vi "ros1.vi"() -> ()   [LabVIEW 2015]
uses:
  <vilib>/Tufts CEEO ROS for LabVIEW Software/ROS/Code/Console/Servers/ServerSubs/TopicDef.ctl
  <vilib>/Tufts CEEO ROS for LabVIEW Software/ROS/Code/SubVIs/_ROSDirection.ctl
  <vilib>/Tufts CEEO ROS for LabVIEW Software/ROS/MessageParsing/std_msgs/subs/parse_bool_scalar.vi
panel:
  out "bool":bool
  in  "Definitions":T1={"Topic"="/robot/head/command_head_nod", "Type"="std_msgs/Bool", "Action"=enum."Publisher", "Update (ms)"=1, "queue size"=1}
  in  "node":string
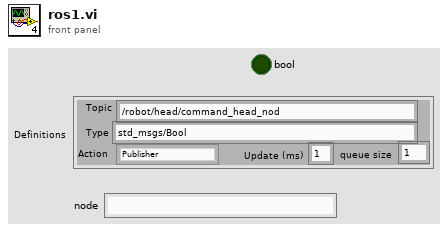
[diagram p1: front panel]
types:
  T1 = typedef "TopicDef.ctl" = cluster{"Topic":string, "Type":string, "Action":T2, "Update (ms)":u16, "queue size":u16}
  T2 = typedef "_ROSDirection.ctl" = enum16{"Node", "Publisher", "Subscriber", "ServiceClient", "ServiceProvider"}
  T3 = typedef "_ROSControl.ctl" = cluster{"topic port":u16, "Node":string, "topic":string, "type":string, "node port":u16, "error ":errorcluster, "Direction":T2, "Update (ms)":u16, "FIFO size":u16}
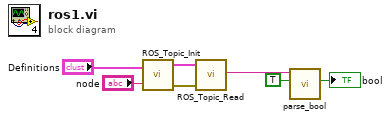
[diagram p0: block diagram]
diagram:
  n1 = call <vilib>:"ROS_Topic_Init.vi"("Definitions"="Definitions", "node"="node") -> ("ROS out"=w4:T3, "error out"=w5:errorcluster)  [unwired: 1 in]
  n2 = call <vilib>:"ROS_Topic_Read.vi"("error in (no error)"=w5, "ROS in"=w4) -> ("Reply"=w3:string)  [unwired: 1 in, 2 out]
  n3 = call-poly <vilib>:"parse_bool.vi"("type"=TRUE, "msg in"=w3) -> ("bool"=→"bool":bool)  [unwired: 3 in, 2 out]
